vi "Input_Roller_Commands.vi"(11 "All Joysticks":T1) -> (3 "Roller Commands":T4)   [LabVIEW 2012]
uses:
  Input_Commands_Roller.ctl
  Input_All_Joysticks.ctl
  Input_Single_Joystick.ctl
  <vilib>/Rock Robotics/WPI/Joystick/WPI_JoystickButtonState.ctl
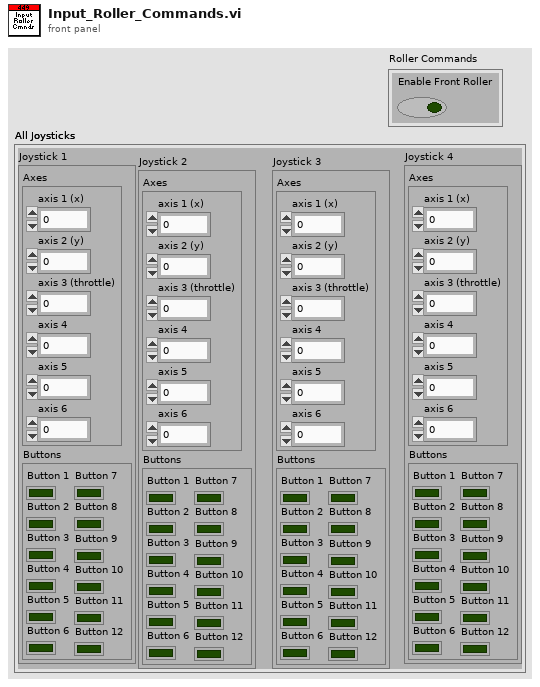
[diagram p1: front panel]
types:
  T1 = typedef "Input_All_Joysticks.ctl" = cluster{"Joystick 1":T2, "Joystick 2":T2, "Joystick 3":T2, "Joystick 4":T2}
  T2 = typedef "Input_Single_Joystick.ctl" = cluster{"Axes":cluster{"axis 1 (x)":dbl, "axis 2 (y)":dbl, "axis 3 (throttle)":dbl, "axis 4":dbl, "axis 5":dbl, "axis 6":dbl}, "Buttons":T3}
  T3 = typedef "WPI_JoystickButtonState.ctl" = cluster{"Button 1":bool, "Button 2":bool, "Button 3":bool, "Button 4":bool, "Button 5":bool, "Button 6":bool, "Button 7":bool, "Button 8":bool, "Button 9":bool, "Button 10":bool, "Button 11":bool, "Button 12":bool}
  T4 = typedef "Input_Commands_Roller.ctl" = cluster{"Enable Front Roller":bool}
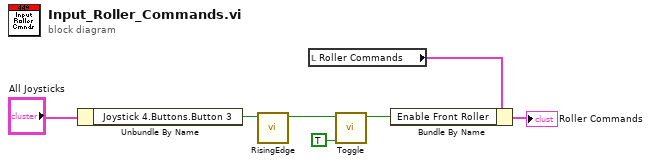
[diagram p0: block diagram]
diagram:
  n1 = Unbundle By Name("All Joysticks") -> ("Joystick 4.Buttons.Button 3"=w2:bool)
  n2 = call "RisingEdge.vi"("BooleanIn"=w2) -> ("BooleanOut"=w1:bool)  [unwired: 10 in]
  n3 = local read "Roller Commands"() -> (w6:T4)
  n4 = call "Toggle.vi"("Initial"=TRUE, "Toggle"=w1) -> ("BoolOut"=w4:bool)  [unwired: 9 in]
  n5 = Bundle By Name(cluster=w6, "Enable Front Roller"=w4) -> (→"Roller Commands":T4)
